vi "ReadDtc.vi"(5 "LogSuspend":bool, 8 "error in":errorcluster, 10 "Paramter":string="02 08", 11 "UdsHandleIn":T1={"LogPath"=path "", "LogEnabled"=FALSE, "isOpen"=FALSE, "LogContent"="", "Adapter"="CAN0", "MCanHandle"={"MCanAdapter"=refnum}, "TransmittId"=0, "ReceiveId"=0}) -> (0 "error out":errorcluster, 1 "DtcItems":T3[](array[typedef]), 2 "DtcLineOut":string, 3 "UdsHandleOut":T1={"LogPath"=path "", "LogEnabled"=FALSE, "isOpen"=FALSE, "LogContent"="", "Adapter"="CAN0", "MCanHandle"={"MCanAdapter"=refnum}, "TransmittId"=0, "ReceiveId"=0})   [LabVIEW 2011, in "Konvolucio MUDS150628.lvlib"]
uses:
  <instrlib>/Konvolucio MUDS150628/Konvolucio MUDS150628.lvlib
  <instrlib>/Konvolucio MUDS150628/Types/DtcItemType.ctl
  <instrlib>/Konvolucio MUDS150628/Types/UdsHandleType.ctl
  <instrlib>/Konvolucio MCAN120803/Types/MCanHandleType.ctl
  C:/Program Files/National Instruments/LabVIEW 2011/instr.lib/Konvolucio MCAN120803/Private/Konvolucio.MCAN120803.dll
  Konvolucio MCAN120803/Private/Konvolucio.MCAN120803.dll
  <instrlib>/Konvolucio MCAN120803/Konvolucio MCAN120803.lvlib
panel:
  out "DtcCount":i32
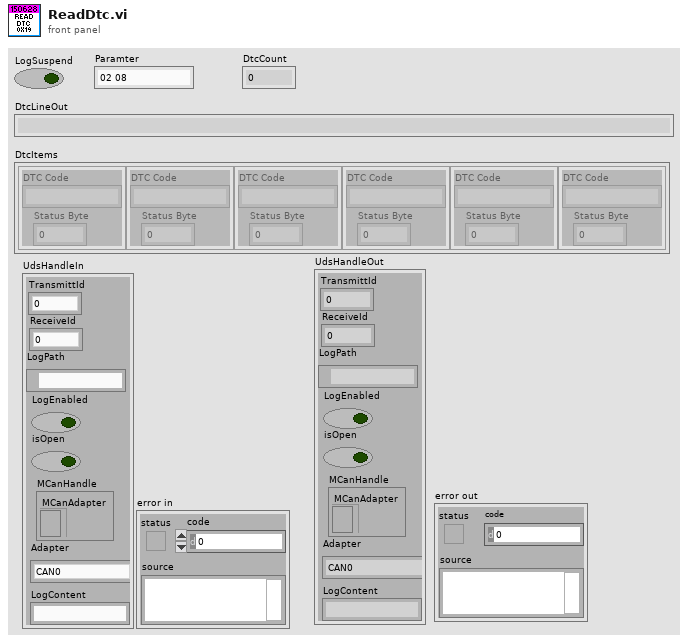
[diagram p1: front panel]
types:
  T1 = typedef "Konvolucio MUDS150628.lvlib/UdsHandleType.ctl" = cluster{"LogPath":path, "LogEnabled":bool, "isOpen":bool, "LogContent":string, "Adapter":string, "MCanHandle":T2, "TransmittId":u32, "ReceiveId":u32}
  T2 = typedef "Konvolucio MCAN120803.lvlib/MCanHandleType.ctl" = cluster{"MCanAdapter":refnum<k24>}
  T3 = typedef "Konvolucio MUDS150628.lvlib/DtcItemType.ctl" = cluster{"DTC Code":string, "Status Byte":i32}
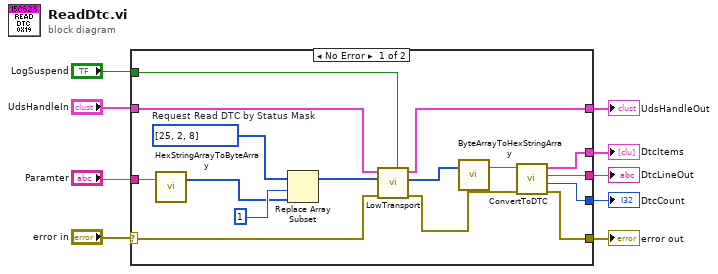
[diagram p0: block diagram]
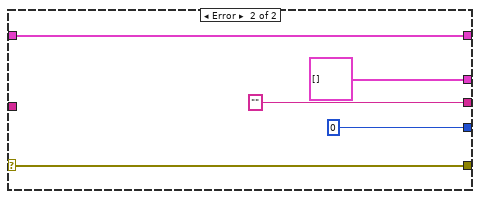
[diagram p2: hidden frame]
diagram:
  n1 = case shown="No Error" "error in" {
    selector: "error in" -> [w20 w27]
    tunnel: [w25 "" ("DtcLineOut")] -> w9
    tunnel: [w24 T3[] [] ("DtcItems")] -> w8
    tunnel: [w22 w27] -> w7
    tunnel: [w18 w30] -> w6
    tunnel: "UdsHandleIn" -> [w21 w30]
    tunnel: "LogSuspend" -> [w19 _]
    tunnel: [w17 0 ("Lenght")] -> w2
    tunnel: "Paramter" -> [w10 _]
    frame No Error {
      w11 = u8[] [25, 2, 8]  # Request Read DTC by Status Mask
      n2 = call <instrlib>:"HexStringArrayToByteArray.vi"("HexStirngArray"=w10) -> ("ByteArrayOut"=w13:u8[])  [unwired: 2 in]
      n3 = Replace Array Subset(array=w11, new element=w13, index=1) -> (w12:u8[])
      n4 = call <instrlib>:"LowTransport.vi"("LogSuspend"=w19, "error in"=w20, "Request"=w12, "HandleIn"=w21) -> ("error out"=w23:errorcluster, "Response"=w15:u8[], "HandleOut"=w18:T1)  [unwired: 5 in]
      n5 = call <instrlib>:"ByteArrayToHexStringArray.vi"("ByteArrayIn"=w15) -> ("HexStringArrayOut"=w16:string)  [unwired: 2 in]
      n6 = call <instrlib>:"ConvertToDTC.vi"("error in"=w23, "DataLineIn"=w16) -> ("error out"=w22:errorcluster, "Lenght"=w17:i32, "DtcLineOut"=w25:string, "DtcItems"=w24:T3[])  [unwired: 6 in]
    }
    frame Error {
    }
  }
  "error out" <- w7
  "DtcLineOut" <- w9
  "DtcItems" <- w8
  "UdsHandleOut" <- w6
  "DtcCount" <- w2
